vi "读取数据库.vi"(7 "condition":string, 8 "error in (no error)":errorcluster caption="错误输入（无错误）", 9 "database":string="database1.mdb", 10 "显示项":string[](array[string]), 11 "组合框":string(combo)) -> (0 "error out":errorcluster caption="错误输出", 1 "columns":string[](array[string]), 2 "data":variant[][](array[variant]), 3 "表格":string[][](table))   [LabVIEW 2016, in "数据查询.lvlib"]
uses:
  <vilib>/addons/database/Connection.llb/DB Tools Open Connec (String).vi
  <vilib>/addons/database/_DB Variant To Data/Database Variant To Data.xnode
  <vilib>/addons/database/NI_Database_API.lvlib
  database/Access/Access Lib.lvlib
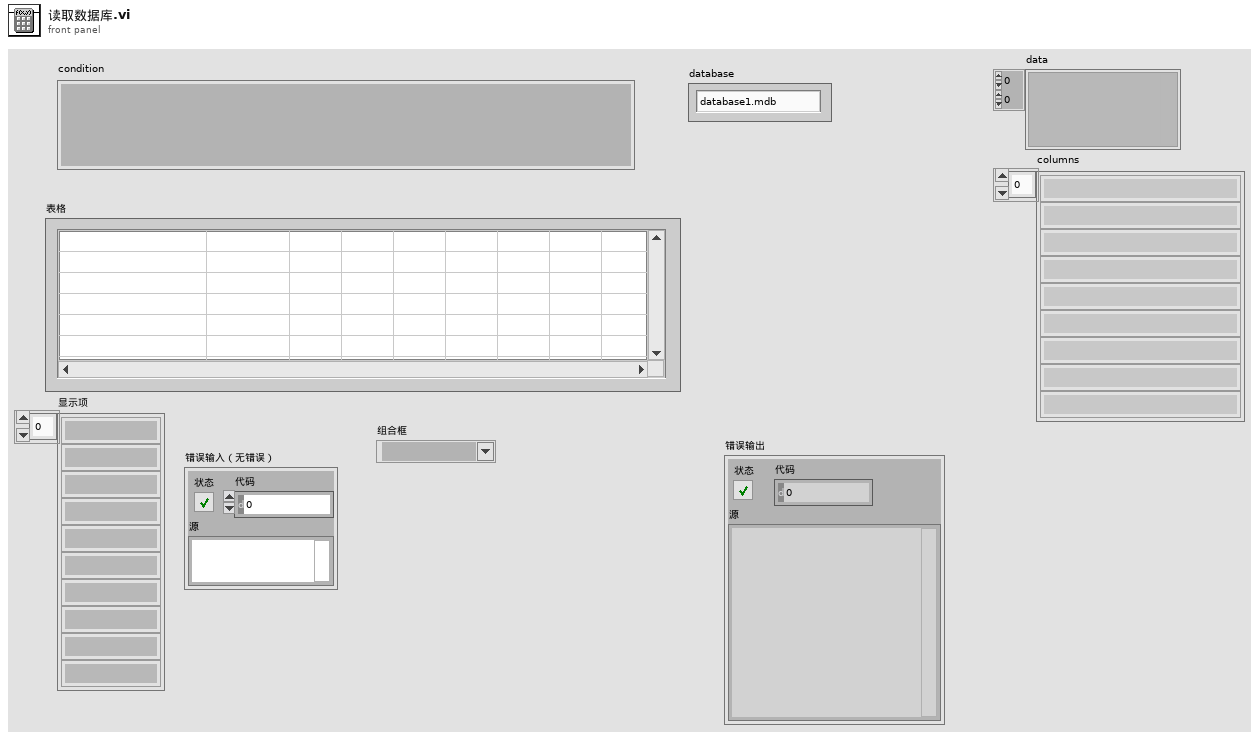
[diagram p1: front panel]
types:
  T1 = typedef "NI_Database_API.lvlib/Conn ObjectReference.ctl" = refnum<k1>
  T2 = typedef "NI_Database_API.lvlib/DB Tools DataTypes.ctl" = enum16{"String", "Long (I32)", "Single (SGL)", "Double (DBL)", "Date/Time", "Binary"}
  T3 = cluster{"name":string, "database data type":T2, "defined size":i32}[]
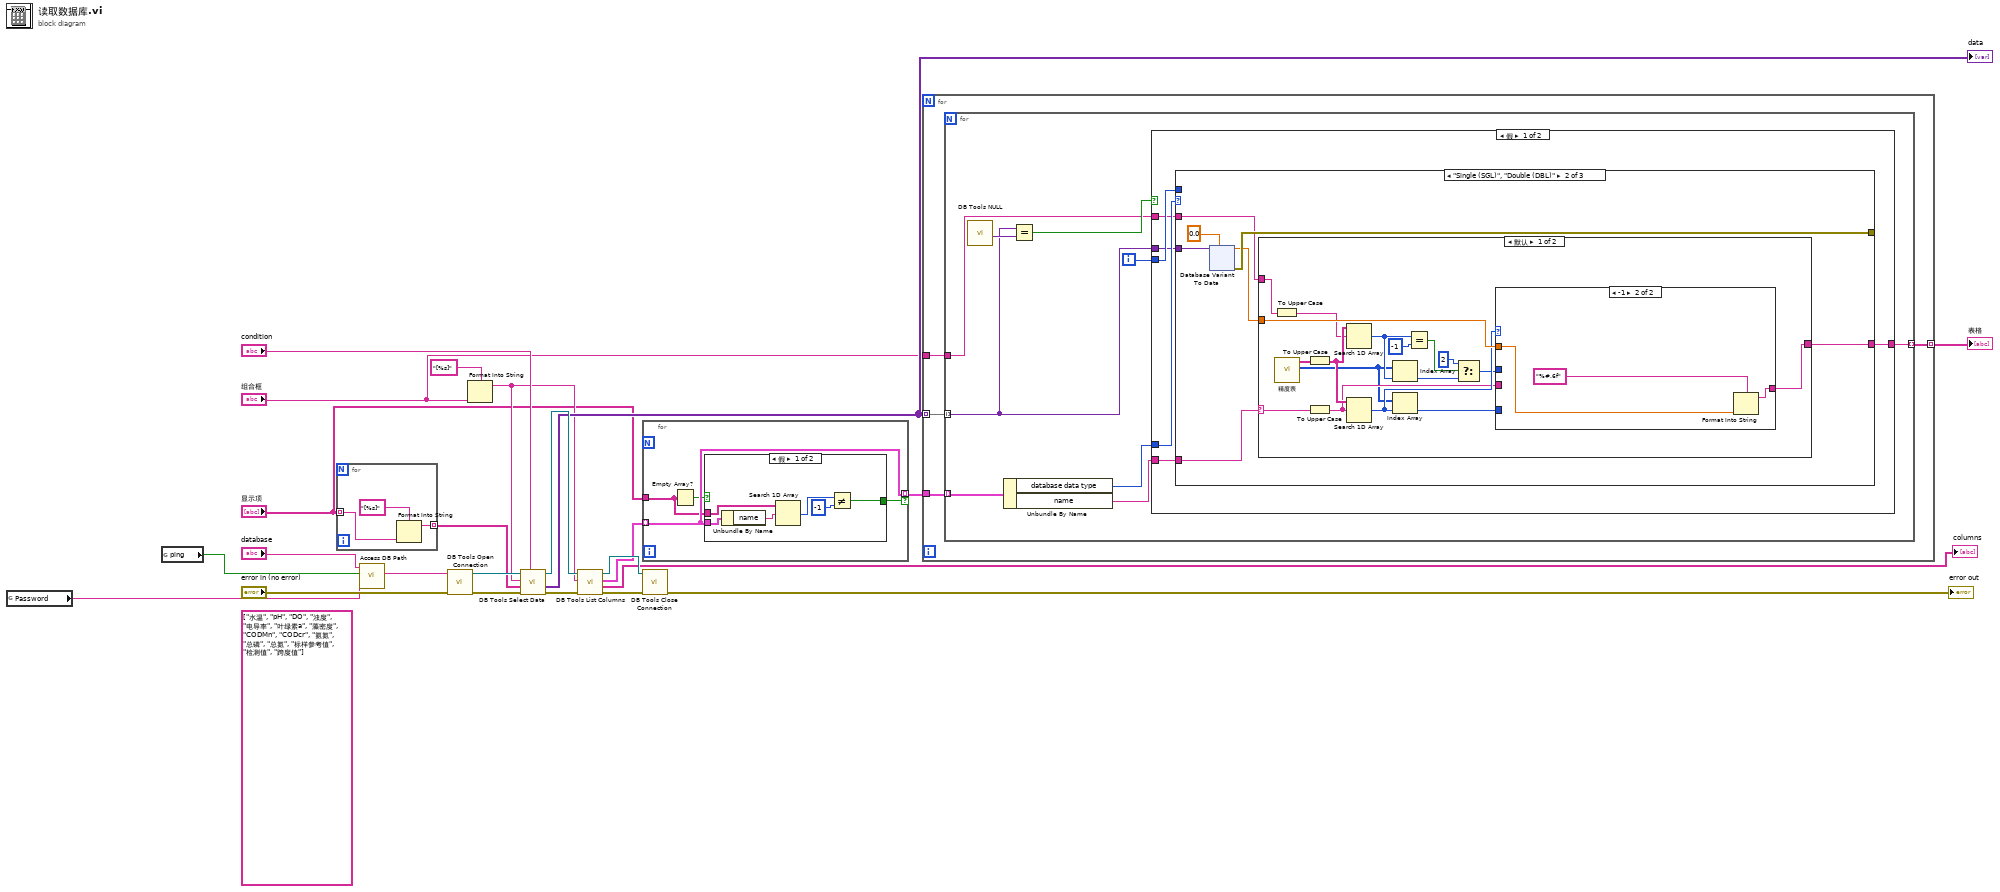
[diagram p0: block diagram]
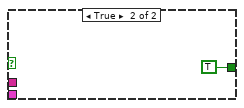
[diagram p2: hidden frame]
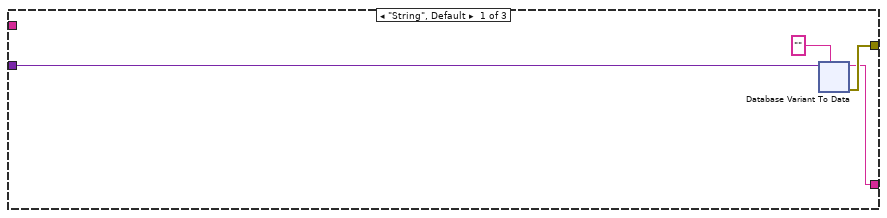
[diagram p3: hidden frame]
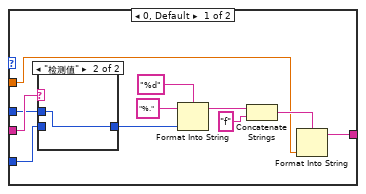
[diagram p4: hidden frame]
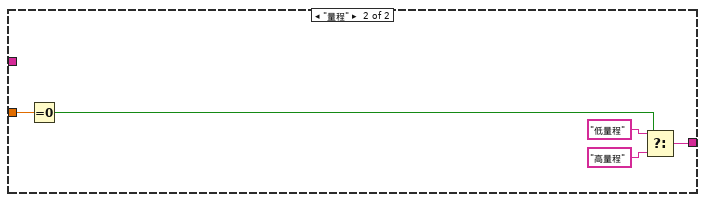
[diagram p6: hidden frame]
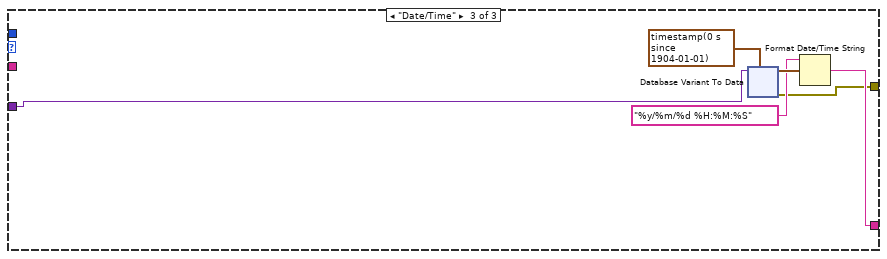
[diagram p7: hidden frame]
diagram:
  (unwired) string[] ["水温", "pH", "DO", "浊度", "电导率", "叶绿素a", "藻密度", "CODMn", "CODcr", "氨氮", "总磷", "总氮", "标样参考值", "检测值", "跨度值"]
  n1 = global read "外部调用接口全局变量.vi" "Password"() -> (w1:string)
  n2 = global read "全局变量.vi" "ping"() -> (w2:bool)
  n3 = for {
    tunnel: "显示项" -> [w26] mode=indexing
    tunnel: [w25] -> w3 mode=indexing
    n4 = Format Into String(format string="[%s]" ("格式字符串"), w26) -> (resulting string=w25:string)  [unwired: 2 in, 1 out]
  }
  n5 = call "Access DB Path.vi"("Password"=w1, "ping"=w2, "database"="database") -> ("Connection information"=w5:string)  [unwired: 7 in, 1 out]
  n6 = call-poly <vilib>:"DB Tools Open Connection.vi"("error in (no error)"="error in (no error)", "connection information"=w5) -> ("error out"=w22:errorcluster, "connection reference"=w23:T1)  [unwired: 6 in]
  n7 = Format Into String(format string="[%s]" ("格式字符串"), "组合框") -> (resulting string=w9:string)  [unwired: 2 in, 1 out]
  n8 = call <vilib>:"DB Tools Select Data.vi"("condition"="condition", "error in (no error)"=w22, "columns"=w3, "table"=w9, "connection reference"=w23) -> ("error out"=w21:errorcluster, "data"=w14:variant[][], "connection reference out"=w18:T1)  [unwired: 1 in]
  "data" <- w14
  n9 = call <vilib>:"DB Tools List Columns.vi"("error in (no error)"=w21, "table"=w9, "connection reference"=w18) -> ("error out"=w15:errorcluster, "columns"=→"columns":string[], "column information"=w11:T3, "connection reference out"=w16:T1)  [unwired: 1 in]
  n10 = for {
    tunnel: w11 -> [w29] mode=indexing
    tunnel: "显示项" -> [w28]
    tunnel: [w29] -> w10 mode=indexing if=w30
    n11 = Empty Array?(array=w28) -> (empty?=w27:bool)
    n12 = case shown="假" w27 {
      tunnel: [w33 TRUE] -> w30
      tunnel: w29 -> [w32 _]
      tunnel: w28 -> [w31 _]
      frame False {
        n13 = Unbundle By Name(w32) -> ("name"=w34:string)
        n14 = Search 1D Array(1D array=w31, element=w34) -> (index of element=w36:i32)  [unwired: 1 in]
        n15 = Not Equal?(x=w36, y=-1) -> (x != y?=w33:bool)
      }
      frame True {
      }
    }
  }
  n16 = call <vilib>:"DB Tools Close Connection.vi"("error in (no error)"=w15, "connection reference"=w16) -> ("error out"=→"error out":errorcluster)  [unwired: 5 in]
  n17 = for {
    tunnel: w14 -> [w41] mode=indexing
    tunnel: w10 -> [w40]
    tunnel: [w39] -> w13 mode=indexing
    tunnel: "组合框" -> [w38]
    n18 = for {
      tunnel: w41 -> [w46] mode=indexing
      tunnel: w40 -> [w50] mode=indexing
      tunnel: [w48] -> w39 mode=indexing
      tunnel: w38 -> [w44]
      i -> [w49]
      n19 = call <vilib>:"DB Tools NULL.vi"() -> ("NULL"=w47:variant)  [unwired: 10 in, 1 out]
      n20 = Unbundle By Name(w50) -> ("database data type"=w43:T2, "name"=w42:string)
      n21 = Equal?(x=w46, y=w47) -> (x = y?=w45:bool)
      n22 = case shown="假" w45 {
        tunnel: w43 -> [w56 _]
        tunnel: w49 -> [w55 _]
        tunnel: [w54 _] -> w48
        tunnel: w42 -> [w53 _]
        tunnel: w46 -> [w52 _]
        tunnel: w44 -> [w51 _]
        frame False {
          n23 = case shown="\"Single (SGL)\", \"Double (DBL)\"" w56 {
            tunnel: w52 -> [w60 w97 w175]
            tunnel: [w57 w98 w171] -> w54
            tunnel: w55 -> [_ _ _]
            tunnel: [w58 w99 w170] -> _
            tunnel: w53 -> [_ w96 _]
            tunnel: w51 -> [_ w93 _]
            frame "String", Default {
              n24 = xnode "Database Variant To Data"("database variant"=w60, "type"="") -> ("data"=w57:string, "error out"=w58:errorcluster)  [unwired: 1 in]
            }
            frame "Single (SGL)", "Double (DBL)" {
              n25 = xnode "Database Variant To Data"("database variant"=w97, "type"=0.0) -> ("data"=w94:dbl, "error out"=w99:errorcluster)  [unwired: 1 in]
              n26 = case shown="默认" w96 {
                selector: w96 -> [w114 _]
                tunnel: w94 -> [w116 w137]
                tunnel: [w115 w133] -> w98
                tunnel: w93 -> [w112 _]
                frame Default {
                  n27 = To Upper Case(1:w112) -> (0:w109:string)
                  n28 = call "精度表.vi"() -> ("精度"=w100:i32[], "参数"=w101:string[])  [unwired: 10 in]
                  n29 = To Upper Case(1:w101) -> (0:w110:string[])
                  n30 = To Upper Case(1:w114) -> (0:w108:string)
                  n31 = Search 1D Array(1D array=w110, element=w109) -> (index of element=w107:i32)  [unwired: 1 in]
                  n32 = Search 1D Array(1D array=w110, element=w108) -> (index of element=w113:i32)  [unwired: 1 in]
                  n33 = Index Array(array=w100, index=w107) -> (element=w104:i32)
                  n34 = Index Array(array=w100, index=w113) -> (element=w111:i32)
                  n35 = Equal?(x=w107, y=-1) -> (x = y?=w105:bool)
                  n36 = Select(t=2, s=w105, f=w104) -> (s? t:f=w103:i32)
                  n37 = case shown="-1" w113 {
                    tunnel: w116 -> [w121 w132]
                    tunnel: [w119 w131] -> w115
                    tunnel: w108 -> [w120 _]
                    tunnel: w103 -> [w118 _]
                    tunnel: w111 -> [w117 _]
                    frame 0, Default {
                      n38 = case shown="\"检测值\"" w120 {
                        tunnel: [w128 w129] -> w127
                        tunnel: w118 -> [_ w129]
                        tunnel: w117 -> [w128 _]
                        frame Default {
                        }
                        frame "检测值" {
                        }
                      }
                      n39 = Format Into String(format string="%d" ("格式字符串"), initial string="%." ("初始字符串"), w127) -> (resulting string=w125:string)  [unwired: 1 in, 1 out]
                      n40 = Concatenate Strings(w125, "f" ("格式字符串")) -> (w123:string)
                      n41 = Format Into String(format string=w123, w121) -> (resulting string=w119:string)  [unwired: 2 in, 1 out]
                    }
                    frame -1 {
                      n42 = Format Into String(format string="%#.6f" ("格式字符串"), w132) -> (resulting string=w131:string)  [unwired: 2 in, 1 out]
                    }
                  }
                }
                frame "量程" {
                  n43 = Equal To 0?(x=w137) -> (x = 0?=w136:bool)
                  n44 = Select(t="低量程" ("格式字符串"), s=w136, f="高量程" ("格式字符串")) -> (s? t:f=w133:string)
                }
              }
            }
            frame "Date/Time" {
              n45 = xnode "Database Variant To Data"("database variant"=w175, "type"=timestamp(0 s since 1904-01-01) ("当前时间")) -> ("data"=w174:timestamp, "error out"=w170:errorcluster)  [unwired: 1 in]
              n46 = Format Date/Time String(time format string (%c)="%y/%m/%d %H:%M:%S" ("时间格式字符串(%c)"), seconds (now)=w174) -> (date/time string=w171:string)  [unwired: 1 in]
            }
          }
        }
        frame True {
        }
      }
    }
  }
  "表格" <- w13
